vi "Roller Intake.vi"(6 "Intake Start":bool, 7 "Shoot":bool, 8 "Abort":bool, 9 "Low Shot":bool, 10 "High Shot":bool, 11 "Ball In Position":bool) -> (0 "Roller Motor Set":dbl, 1 "Shooter Motor Set":dbl, 2 "Arm Down":bool, 3 "Ball Ready?":bool)   [LabVIEW 2015]
uses:
  Roller Intake.ctl
panel:
  out "Enum":T1
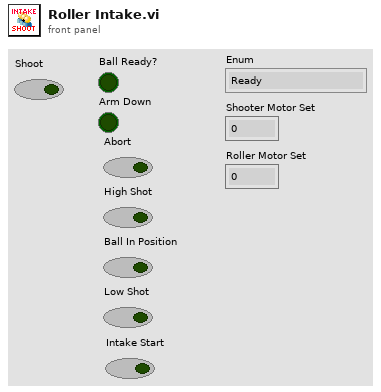
[diagram p1: front panel]
types:
  T1 = typedef "Roller Intake.ctl" = enum16{"Ready", "Intaking", "Ball Set in Position", "Ready to Shoot", "High Shot Preparation", "High Shot", "Low Shot"}
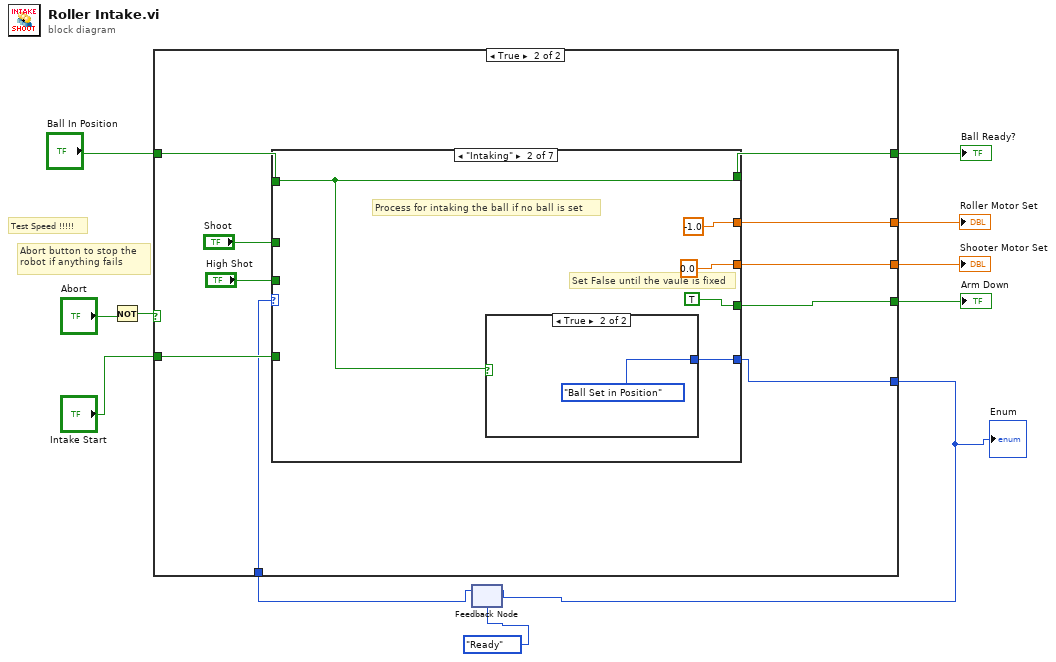
[diagram p0: block diagram]
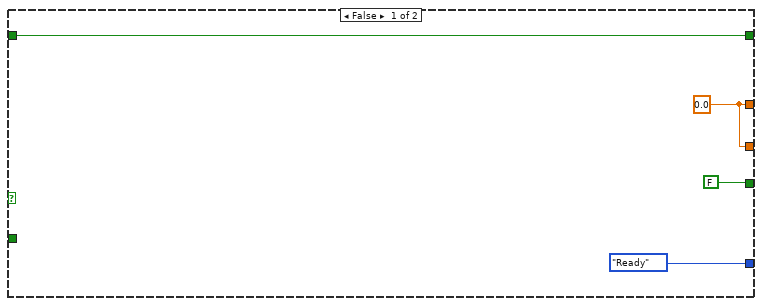
[diagram p2: hidden frame]
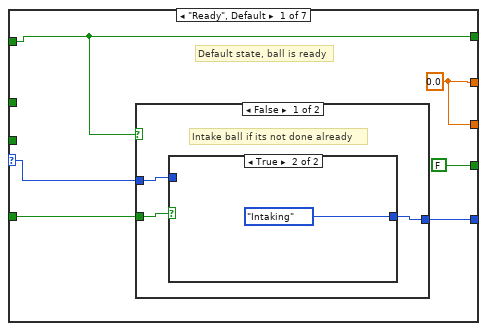
[diagram p3: hidden frame]
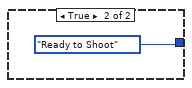
[diagram p5: hidden frame]
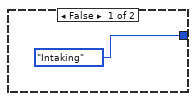
[diagram p6: hidden frame]
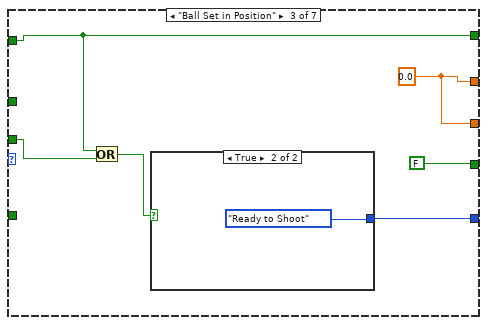
[diagram p7: hidden frame]
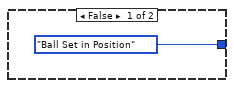
[diagram p8: hidden frame]
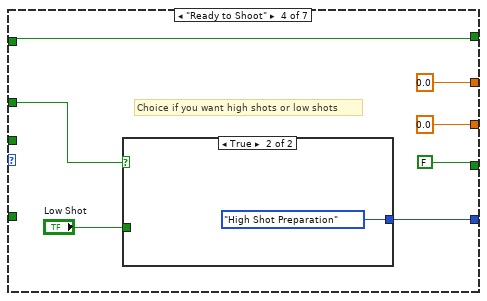
[diagram p9: hidden frame]
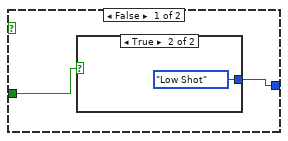
[diagram p10: hidden frame]
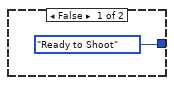
[diagram p11: hidden frame]
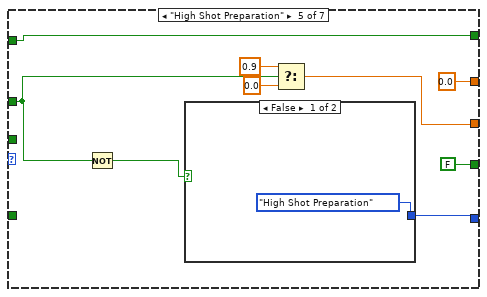
[diagram p12: hidden frame]
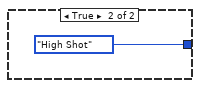
[diagram p13: hidden frame]
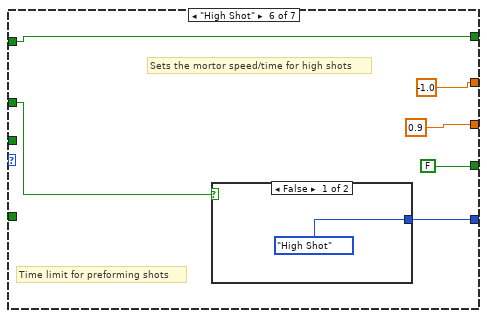
[diagram p14: hidden frame]
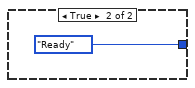
[diagram p15: hidden frame]
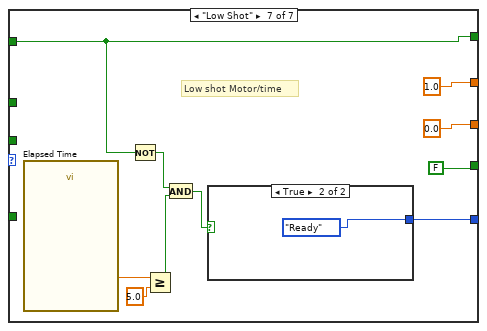
[diagram p16: hidden frame]
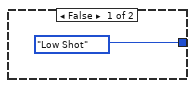
[diagram p17: hidden frame]
diagram:
  # "Test Speed !!!!!"
  # "Abort button to stop the\nrobot if anything fails"
  n1 = Not(x="Abort") -> (.not. x?=w5:bool)
  n2 = feedback #1(Roller_Intake."Ready") -> (w2:T1)
  n3 = case shown="True" w5 {
    tunnel: [w15 w25] -> w11
    tunnel: [w14 w24] -> w10
    tunnel: [FALSE w23] -> w9
    tunnel: [w14 w22] -> w8
    tunnel: "Ball In Position" -> [w15 w18]
    tunnel: "Intake Start" -> [_ w21]
    tunnel: w2 -> [_ w20]
    tunnel: [Roller_Intake."Ready" w19] -> w1
    frame False {
      w14 = 0.0
    }
    frame True {
      n4 = case shown="\"Intaking\"" w20 {
        selector: w20 -> [w27 _ _ _ _ _ _]
        tunnel: [w31 w42 w50 w58 w72 w80 w92] -> w19
        tunnel: [w29 -1.0 w48 0.0 0.0 -1.0 1.0] -> w24
        tunnel: [w26 w40 w47 w59 w73 w79 w91] -> w25
        tunnel: w18 -> [w26 w40 w47 w59 w73 w79 w91]
        tunnel: [FALSE TRUE FALSE FALSE FALSE FALSE FALSE] -> w23
        tunnel: [w29 0.0 w48 0.0 w65 0.9 0.0] -> w22
        tunnel: w21 -> [w28 _ _ _ _ _ _]
        tunnel: "High Shot" -> [_ _ w46 _ _ _ _]
        tunnel: "Shoot" -> [_ _ _ w53 w68 w76 _]
        frame "Ready", Default {
          w29 = 0.0
          # "Default state, ball is ready"
          n5 = case shown="False" w26 {
            tunnel: [w34 Roller_Intake."Ready to Shoot"] -> w31
            tunnel: w28 -> [w33 _]
            tunnel: w27 -> [w32 _]
            frame False {
              # "Intake ball if its not done already"
              n6 = case shown="True" w33 {
                tunnel: [w35 Roller_Intake."Intaking"] -> w34
                tunnel: w32 -> [w35 _]
                frame False {
                }
                frame True {
                }
              }
            }
            frame True {
            }
          }
        }
        frame "Intaking" {
          # "Set False until the vaule is fixed"
          # "Process for intaking the ball if no ball is set"
          n7 = case shown="True" w40 {
            tunnel: [Roller_Intake."Intaking" Roller_Intake."Ball Set in Position"] -> w42
            frame False {
            }
            frame True {
            }
          }
        }
        frame "Ball Set in Position" {
          w48 = 0.0
          n8 = Or(x=w47, y=w46) -> (x .or. y?=w45:bool)
          n9 = case shown="True" w45 {
            tunnel: [Roller_Intake."Ball Set in Position" Roller_Intake."Ready to Shoot"] -> w50
            frame False {
            }
            frame True {
            }
          }
        }
        frame "Ready to Shoot" {
          # "Choice if you want high shots or low shots"
          n10 = case shown="True" w53 {
            tunnel: [w60 Roller_Intake."High Shot Preparation"] -> w58
            tunnel: "Low Shot" -> [w61 _]
            frame False {
              n11 = case shown="True" w61 {
                tunnel: [Roller_Intake."Ready to Shoot" Roller_Intake."Low Shot"] -> w60
                frame False {
                }
                frame True {
                }
              }
            }
            frame True {
            }
          }
        }
        frame "High Shot Preparation" {
          n12 = Not(x=w68) -> (.not. x?=w69:bool)
          n13 = case shown="False" w69 {
            tunnel: [Roller_Intake."High Shot Preparation" Roller_Intake."High Shot"] -> w72
            frame False {
            }
            frame True {
            }
          }
          n14 = Select(t=0.9, s=w68, f=0.0) -> (s? t:f=w65:dbl)
        }
        frame "High Shot" {
          # "Time limit for preforming shots"
          # "Sets the mortor speed/time for high shots"
          n15 = case shown="False" w76 {
            tunnel: [Roller_Intake."High Shot" Roller_Intake."Ready"] -> w80
            frame False {
            }
            frame True {
            }
          }
        }
        frame "Low Shot" {
          # "Low shot Motor/time"
          n16 = call "Elapsed Time"() -> ("Elapsed Time (s)"=w88:dbl)  [unwired: 12 in, 7 out]
          n17 = Not(x=w91) -> (.not. x?=w90:bool)
          n18 = Greater Or Equal?(x=w88, y=5.0) -> (x >= y?=w86:bool)
          n19 = And(x=w90, y=w86) -> (x .and. y?=w89:bool)
          n20 = case shown="True" w89 {
            tunnel: [Roller_Intake."Low Shot" Roller_Intake."Ready"] -> w92
            frame False {
            }
            frame True {
            }
          }
        }
      }
    }
  }
  "Ball Ready?" <- w11
  "Roller Motor Set" <- w10
  "Arm Down" <- w9
  "Shooter Motor Set" <- w8
  "Enum" <- w1
  n21 = feedback-in #1(w1) -> ()
